vi "rqcAlice Key Distribution (Low Level Example).vi"() -> ()   [LabVIEW 2019]
uses:
  Custom Controls/rqcAlice States.ctl
  FPGA/Alice/Custom Controls/Phase Modulator/rqcAlice Mod.Config.ctl
  Shared/Shared FPGA Lib/Shared Logic/Custom Controls/rqc Random Generator.parameters.ctl
  Shared/Shared FPGA Lib/Shared Logic/Custom Controls/rqc Random Generator.value type.ctl
  FPGA/Alice/Custom Controls/Main State Machine/rqcAlice DAC Clock Positions.ctl
  Shared/Shared Host Lib/rqc ServiceNET/Custom Controls/rqc ServiceNET command.ctl
  Shared/Shared Host Lib/rqc ServiceNET/Alice/Custom Controls/rqcAlice ServiceNET control.ctl
  <vilib>/FPGAPlugInAG/PCIe-7820R/niLvFpga_Open_PCIe-7820R.vi
  <vilib>/rvi/interface/common/dynamic/niFpgaDynamicAddResources.vi
  <vilib>/FPGAPlugInAG/Dynamic/niLvFpga_Close_Dynamic.vi
  <vilib>/rvi/interface/nirviOpenFPGA/nirviOpenFPGA.xnode
  FPGA Bitfiles/rqcAlice FPGA (7820R) v 3.2.0.lvbitx
  <vilib>/rvi/interface/nirviCloseFPGA/nirviCloseFPGA.xnode
panel:
  in  "Attenuation, dB":dbl=10.0 max=40.0
  in  "Activate advanced parameters":bool
  in  "Sync mode":bool caption="«Coax / SD»"
  in  "PM RND":bool=TRUE caption="Alice's states randomisation"
  in  "Autoscale X":bool=TRUE caption="Show all QBER mesurements"
  out "QBER Graph":dbl(graph)=3.273809523809524
  out "IP Address":string="192.168.0.245" caption="Alice IP address"
  in  "DL SD":u32 caption="SD delay value"
  in  "pm.off":u8=1
  in  "pm.on":u8=9
  in  "Pi Voltage":u16=130
  out "Real pulse count:":i32=1000000 caption="Real sync pulses count:"
  out "Total pulses expected:":u32=1000000 caption="Sync pulses expected:"
  out "QBER, %":dbl=3.273809523809524
  out "Bob's Key:":string="010101101101101010110001010110000011111000011110110011101010000011100100011000000101000011010101100000000111001111111110010001000100001001000100101010000110100001001101001101100101111010101101000010110000010000000001000010001111000010111000011001111110111101100100010000011110101100100011100000100010001100000001100101100101001001100011001011010110001010010100111010111110001101000001001111101000001010001110011110101110100101011001101000000000101111011111010001001100001100110101000000100000010001001001011101101110100110111101000101110110001101011110011010001000111111101000100000011010000000000100..."
  out "Alice's Key:":string="010101101101101010110001010110000011111000011111110011101010000011100100100000000101000011010101100000000110001111110110000001000100001001000100001010100110100001001101001111100101111110101101000010110000010000000001000010001111000010111000011001111110111101100100010000011110101101100011100000100010001100000001100101100101001001100011001011010110001010010100111010111110101101000001001111101000001010001110011110100110100101011001101000000000101111011111010001001100001100110101000000100000010001001001011101001110000110111101000101110110000101011110011010001000111111101000100000011010000000000100..."
  in  "Pulses in Train":u32=1000 caption="Number of pulses in train"
  in  "Train Number":i32=1000 caption="Number of trains"
  in  "DL Coax":u32=23944 caption="Coax delay value"
  out "error out":errorcluster
  in  "Stop":bool
  out "Connection status":bool
  in  "Port":u16=5020
  out "Current State":T1=enum."App.Stop" caption="App current state"
  # "ALICE"
  # "LAN settings:"
  # "Sync pulses details:"
  # "«"
  # "»"
  # "Advanced\nPM parameters:\nRecommended \npm.on - [9]\npm.off - [1-2]"
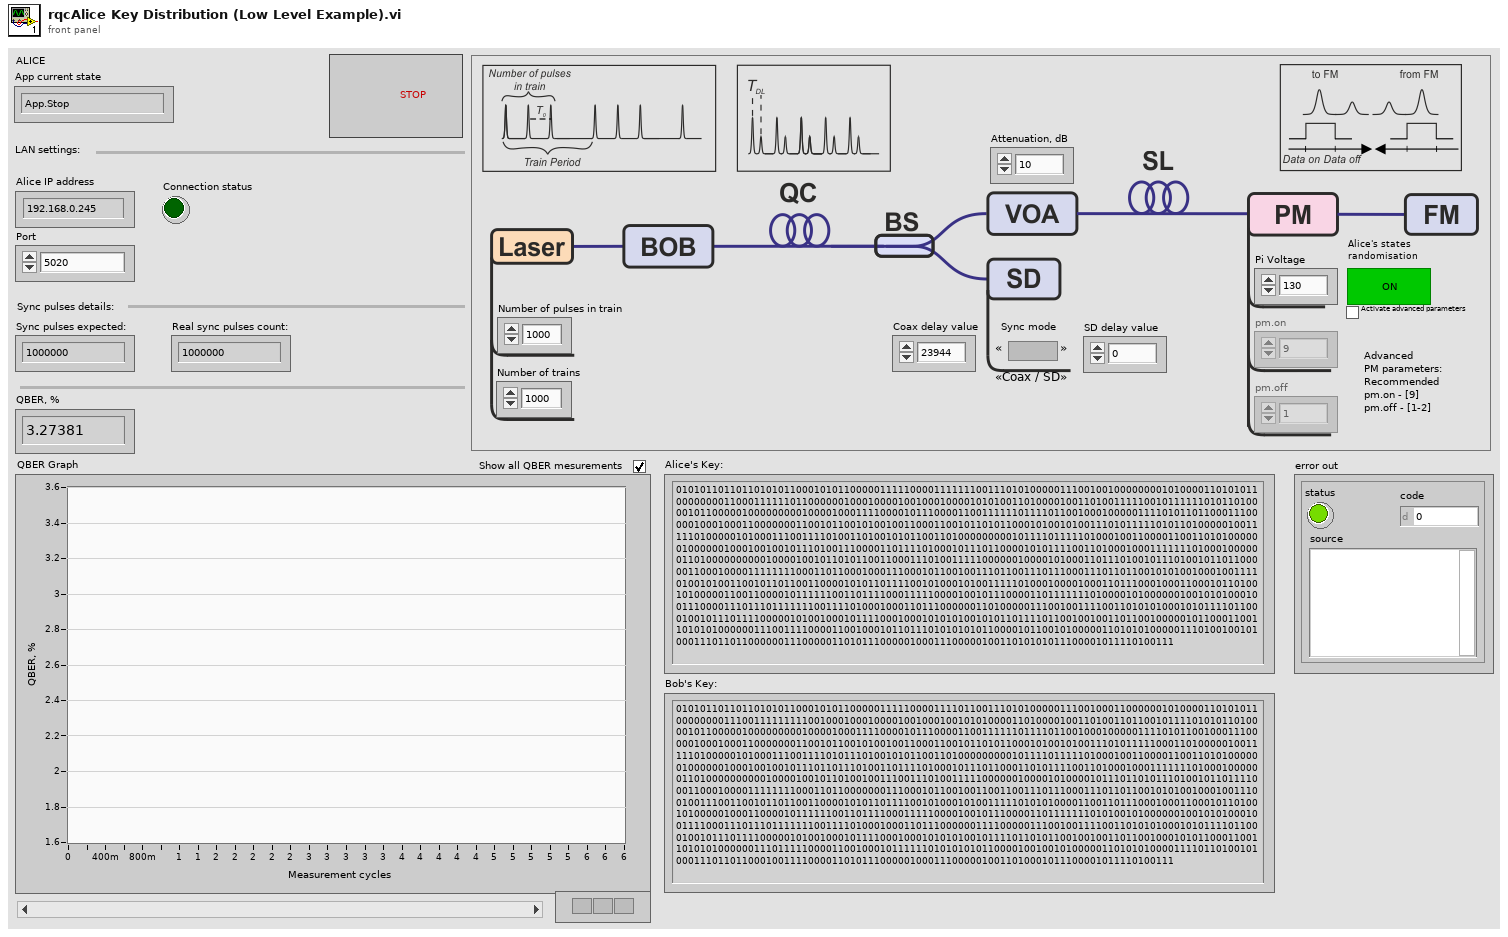
[diagram p1: front panel]
types:
  T1 = typedef "rqcAlice States.ctl" = enum16{"HW.configure", "HW.meas", "NET.create", "NET.connect", "NET.readCommand", "NET.sendCommand", "NET.readData", "NET.close", "Meas.Start", "Meas.NextStep", "Meas.restart", "Meas.Done", "App.HandleEvent", "App.HandleError", "App.Stop"}
  T2 = typedef "rqcAlice DAC Clock Positions.ctl" = u8[]
  T3 = typedef "rqc Random Generator.parameters.ctl" = cluster{"value type":T4, "constant":u16, "num of levels":u16, "levels values":u16[]}
  T4 = typedef "rqc Random Generator.value type.ctl" = enum32{"random value", "constant"}
  T5 = typedef "rqcAlice Mod.Config.ctl" = cluster{"mod.on":u8, "mod.off":u8}
  T6 = typedef "rqc ServiceNET command.ctl" = enum8{"NONE", "READY", "START", "PING"}
  T7 = enum16{"open", "replace", "create", "open or create", "replace or create", "replace or create with confirmation"}
  T8 = typedef "rqcAlice ServiceNET control.ctl" = cluster{"connection ID":refnum<k5>, "port":u16, "connected?":bool}
  T9 = enum8{"Enabled", "Disabled", "Disabled and Grayed Out"}
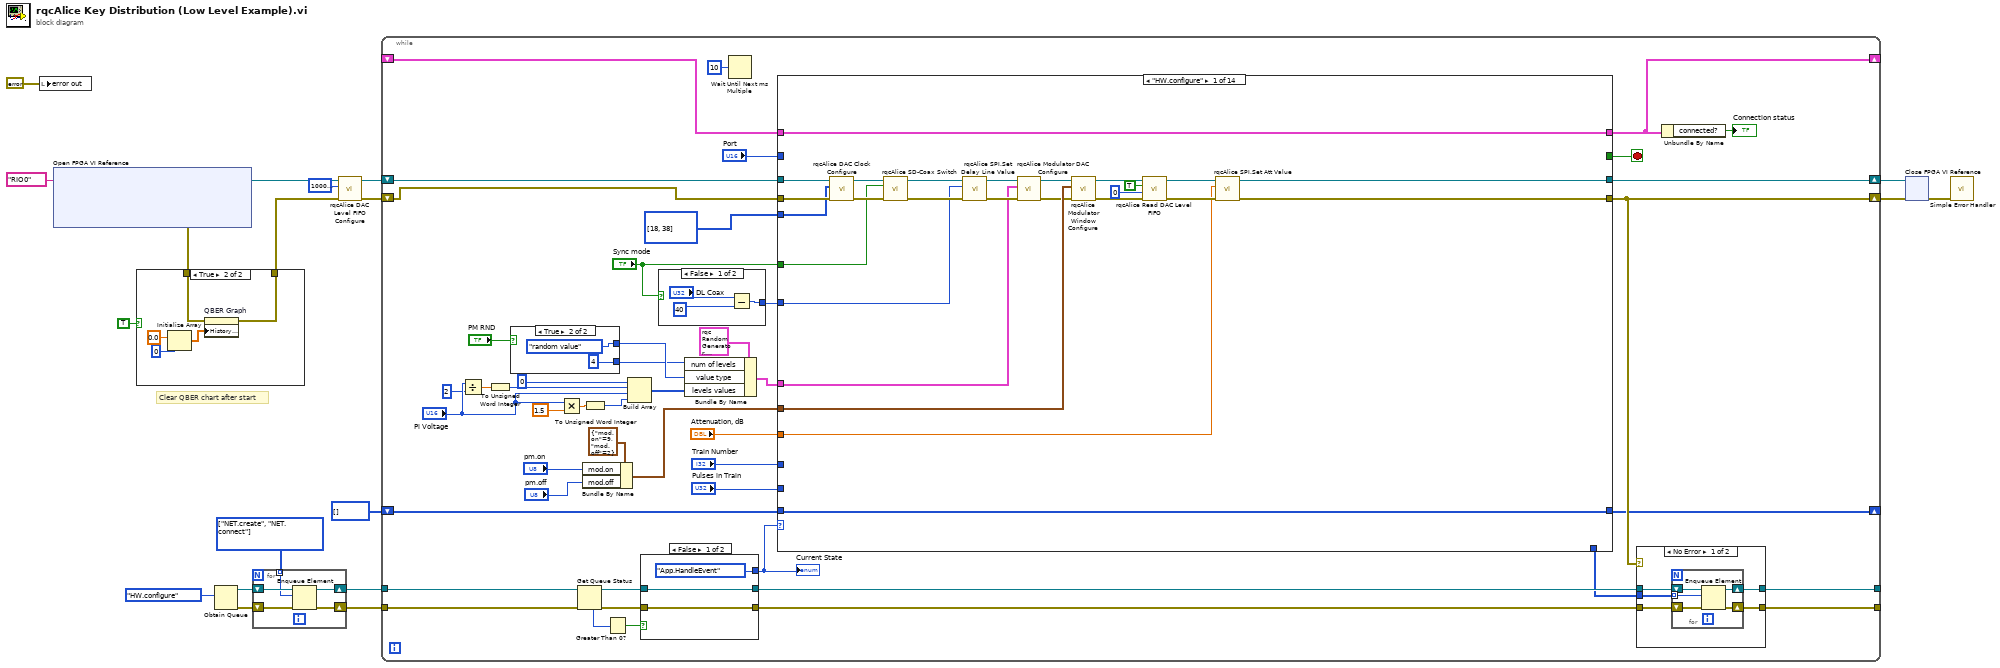
[diagram p0: block diagram]
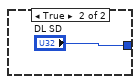
[diagram p3: hidden frame]
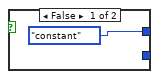
[diagram p4: hidden frame]
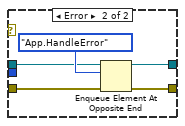
[diagram p5: hidden frame]
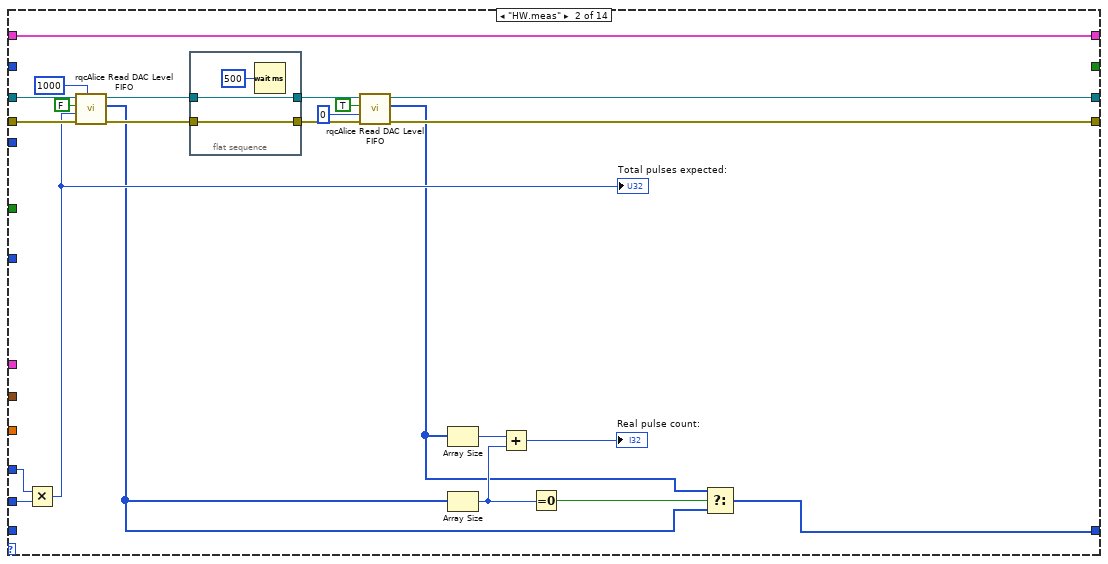
[diagram p6: hidden frame]
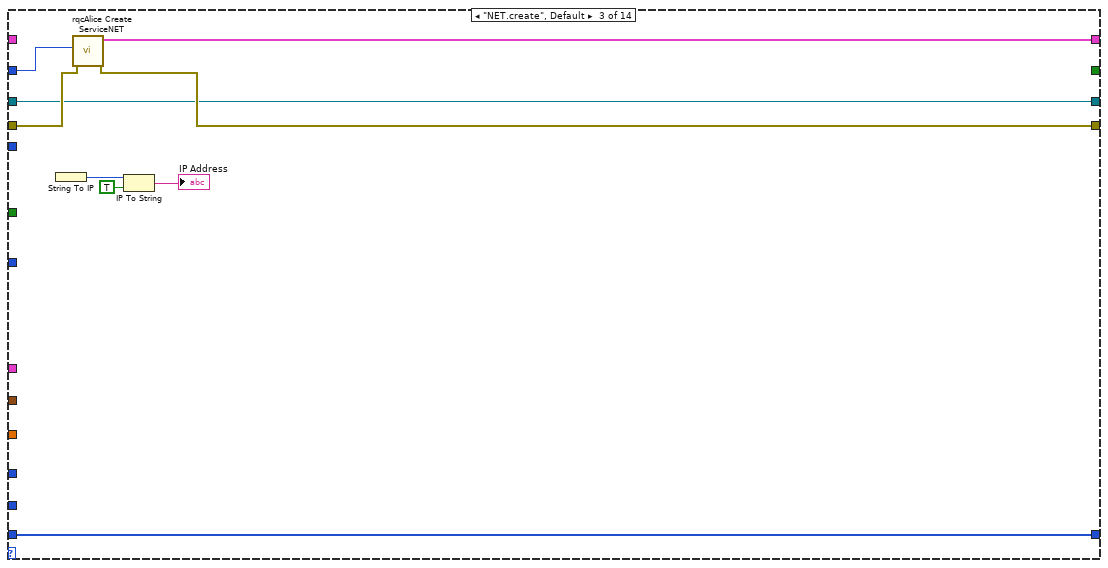
[diagram p7: hidden frame]
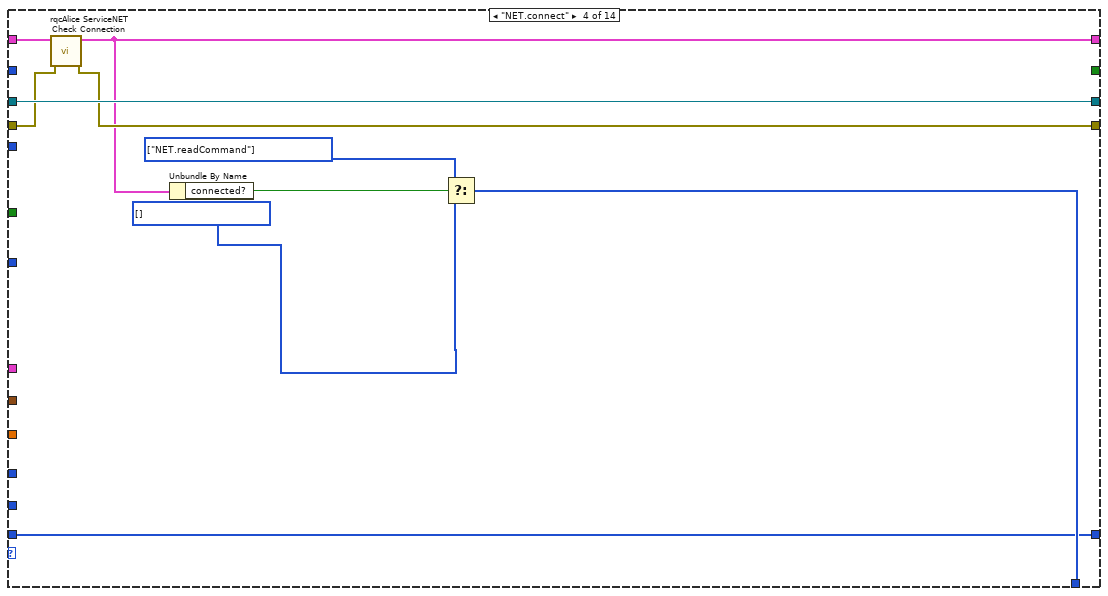
[diagram p8: hidden frame]
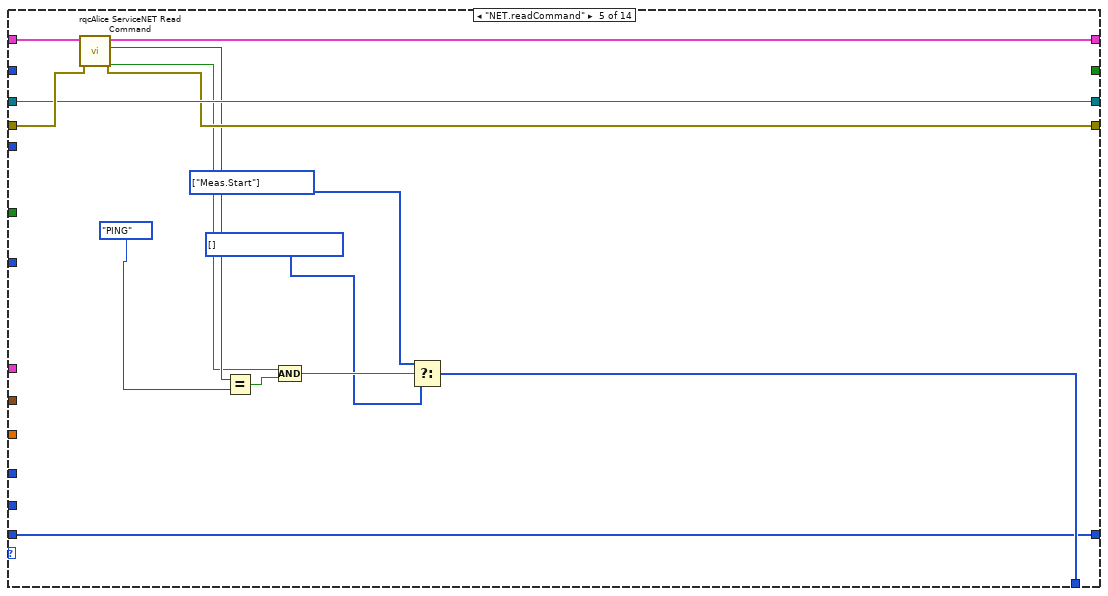
[diagram p9: hidden frame]
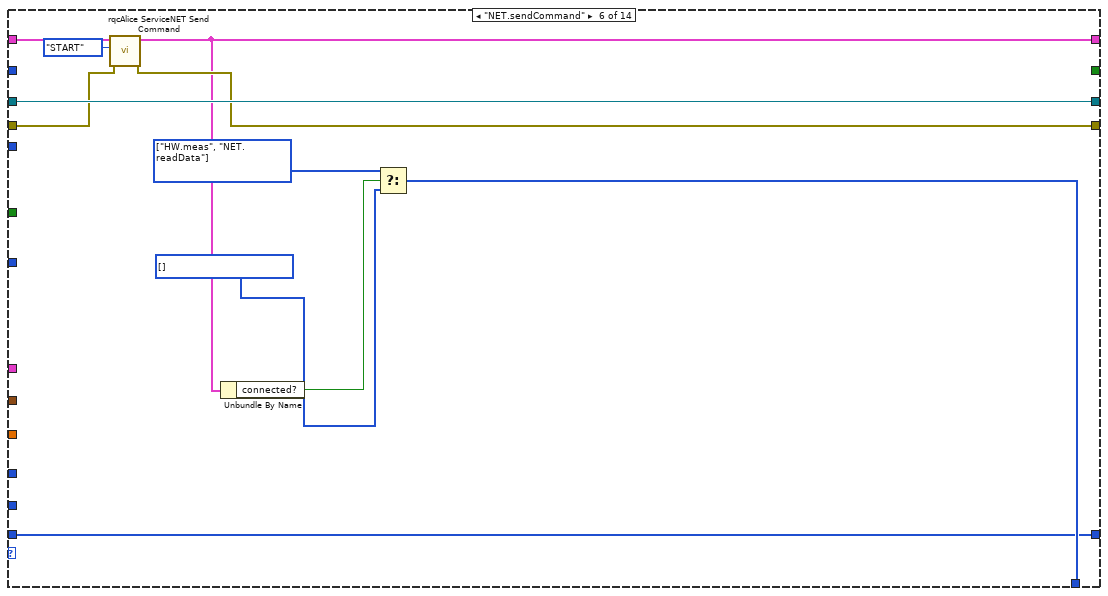
[diagram p10: hidden frame]
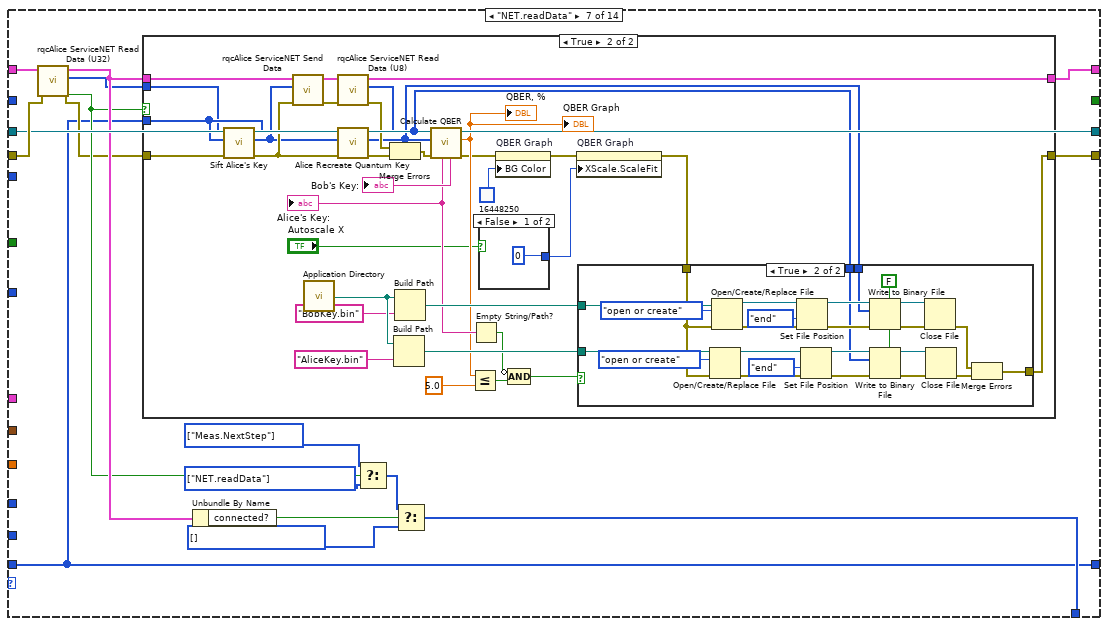
[diagram p11: hidden frame]
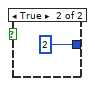
[diagram p13: hidden frame]
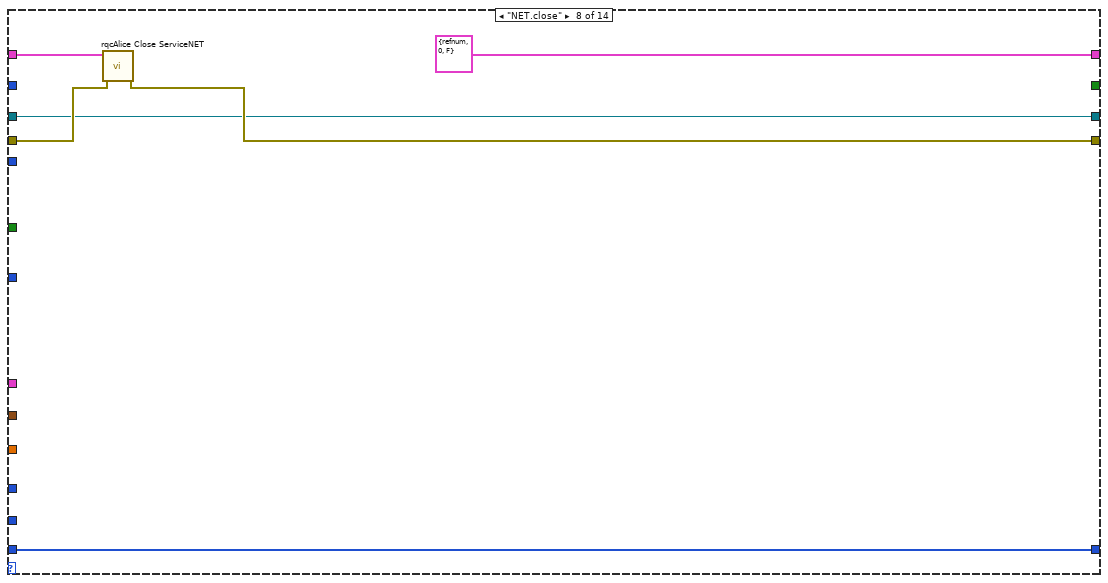
[diagram p15: hidden frame]
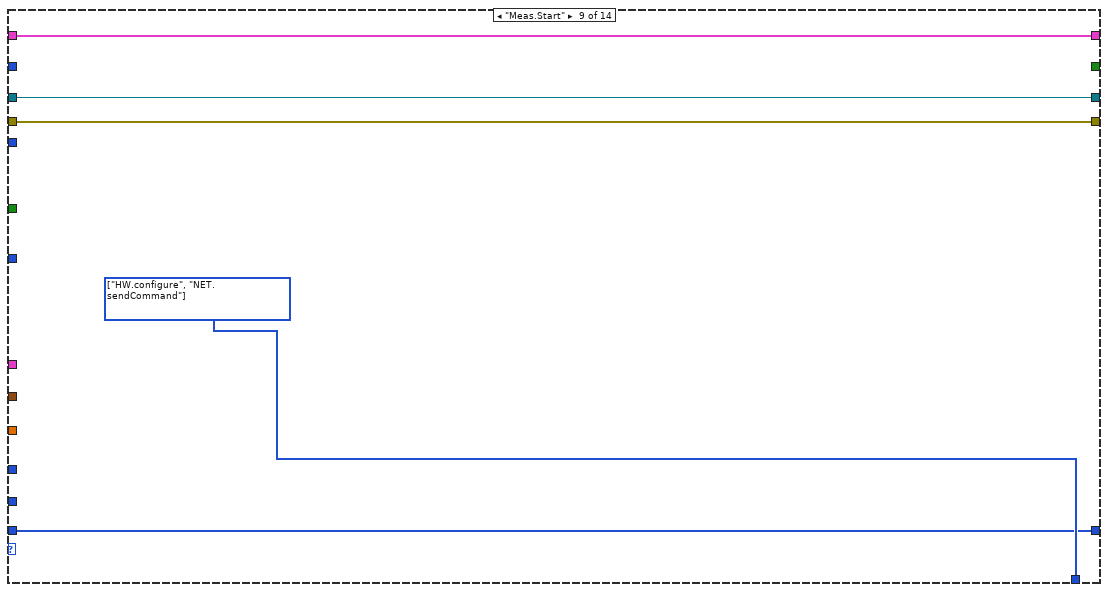
[diagram p16: hidden frame]
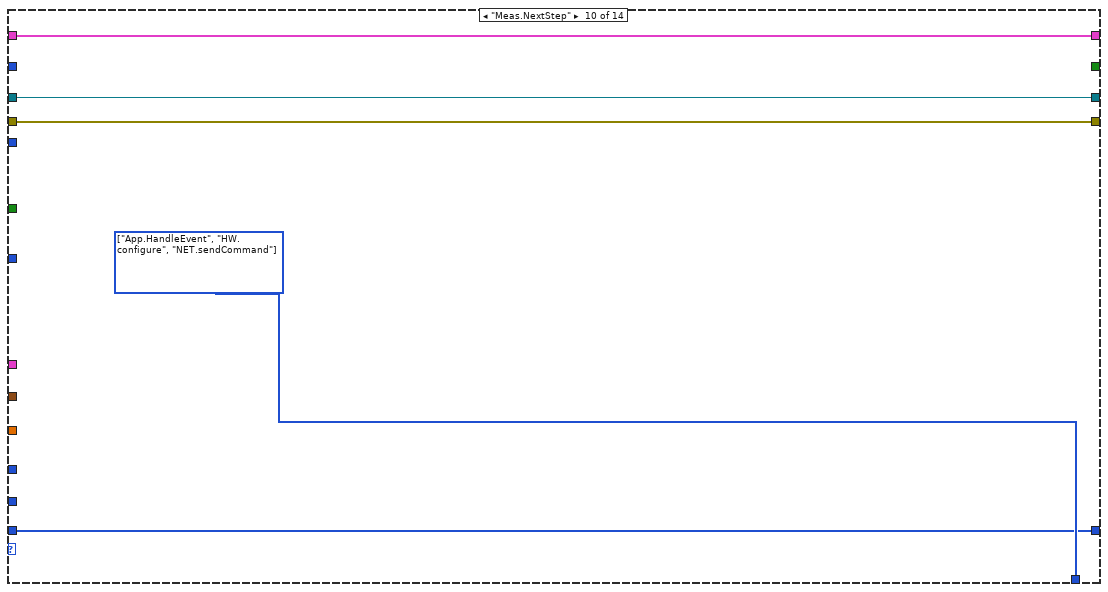
[diagram p17: hidden frame]
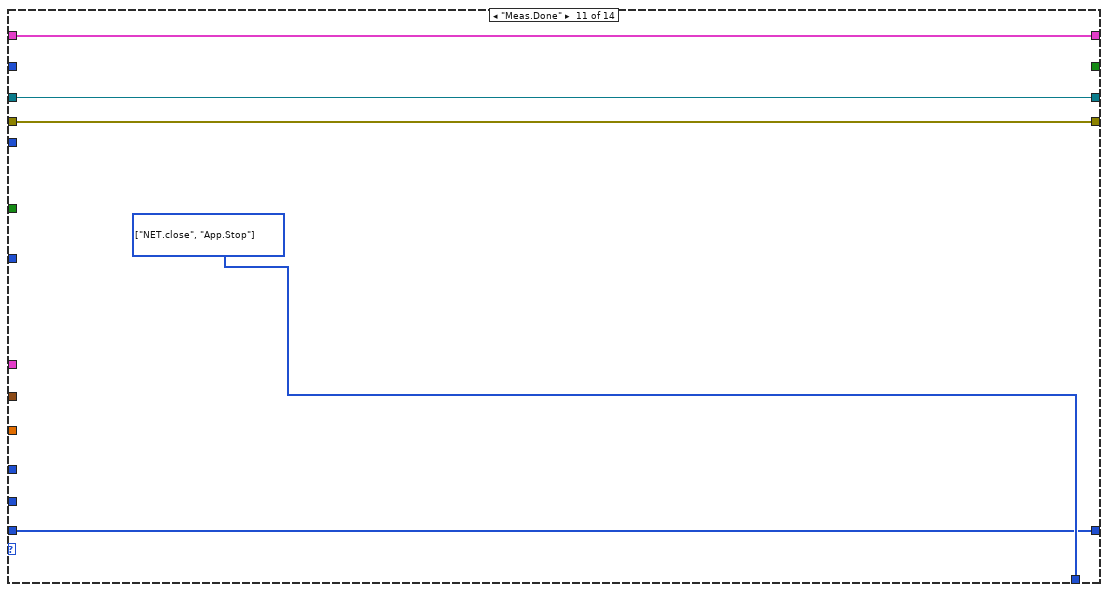
[diagram p18: hidden frame]
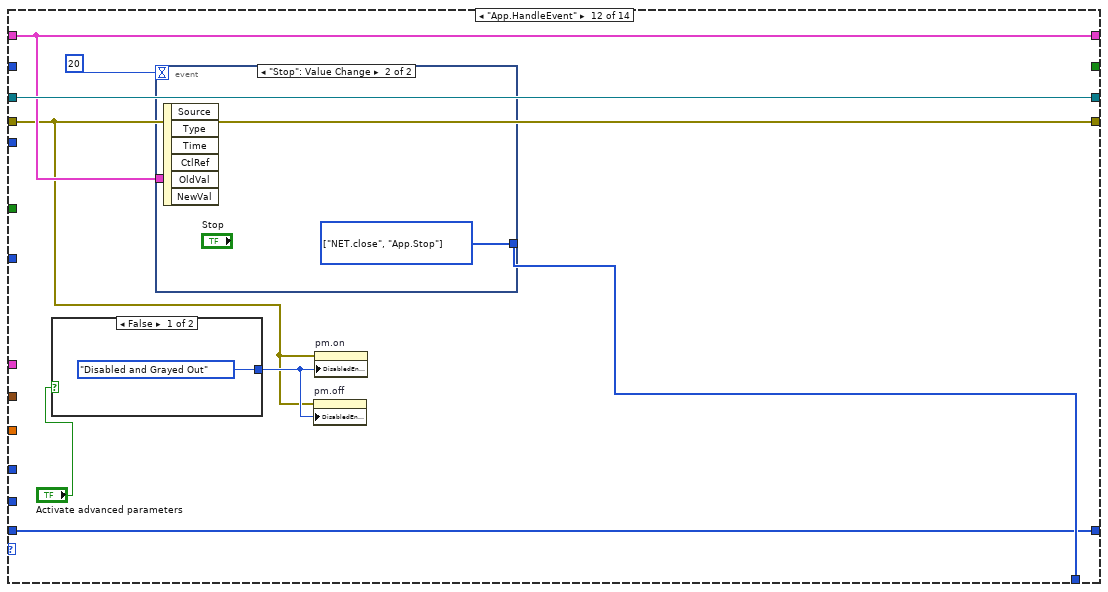
[diagram p19: hidden frame]
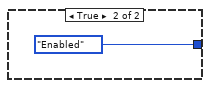
[diagram p20: hidden frame]
diagram:
  w13 = T1[] [enum."NET.create", enum."NET.connect"] items=["HW.configure", "HW.meas", "NET.create", "NET.connect", "NET.readCommand", "NET.sendCommand", "NET.readData", "NET.close", "Meas.Start", "Meas.NextStep", "Meas.restart", "Meas.Done", "App.HandleEvent", "App.HandleError", "App.Stop"]
  # "Clear QBER chart after start"
  n1 = local write "error out"(errorcluster {"status"=FALSE, "code"=0, "source"=""} ("error out")) -> ()
  n2 = xnode "Open FPGA VI Reference"("resource name"=tag "RIO0") -> ("FPGA VI Reference Out"=w8:refnum<k20>, "error out"=w3:errorcluster)  [unwired: 1 in]
  n3 = case shown="True" TRUE {
    tunnel: w3 -> [w20 w25]
    tunnel: [w20 w24] -> w2
    frame False {
    }
    frame True {
      n4 = Initialize Array(0.0 ("element"), 0 ("dimension size")) -> (w23:dbl[])
      n5 = property on="QBER Graph" class="WFChart (strict)"(error in=w25, "History Data"=w23) -> (error out=w24:errorcluster)  [unwired: 1 in, 1 out]
    }
  }
  n6 = Obtain Queue(element data type=rqcAlice_States."HW.configure" ("rqcAlice States")) -> (queue out=w15:refnum<queue>, error out=w14:errorcluster)  [unwired: 4 in, 1 out]
  n7 = for {
    shift-right: [w28] -> w12
    shift-left: w15 -> [w30]
    shift-right: [w27] -> w11
    shift-left: w14 -> [w29]
    tunnel: w13 -> [w26] mode=indexing
    n8 = Enqueue Element(queue=w30, element=w26, error in (no error)=w29) -> (queue out=w28:refnum<queue>, error out=w27:errorcluster)  [unwired: 1 in, 1 out]
  }
  n9 = call "rqcAlice DAC Level FIFO Configure.vi"("error in"=w2, "DAC Level FIFO Depth"=u32 10000000, "Alice FPGA Reference In"=w8) -> ("error out"=w6:errorcluster, "Alice FPGA Reference Out"=w7:refnum<k20>)  [unwired: 7 in]
  n10 = while {
    tunnel: w12 -> [w77]
    shift-right: [w78] -> w18
    shift-left: w7 -> [w41]
    shift-right: [w70] -> w17
    shift-left: w6 -> [w40]
    tunnel: w11 -> [w76]
    tunnel: [w67] -> _
    tunnel: [w66] -> _
    shift-right: [w62] -> _
    shift-left: _ -> [w64]
    shift-right: [w56] -> _
    shift-left: u8[] [] ("Data") -> [w55]
    stop <- w60 stop-if-true
    n11 = Divide(x="Pi Voltage", y=2) -> (x/y=w47:dbl)
    n12 = To Unsigned Word Integer(number=w47) -> (unsigned 16bit integer=w52:u16)
    n13 = case shown="True" "PM RND" {
      tunnel: [rqc_Random_Generator.value_type."constant" ("pm.value type") rqc_Random_Generator.value_type."random value" ("pm.value type")] -> w46
      tunnel: [_ u16 4 ("num of levels")] -> w33
      frame False {
      }
      frame True {
      }
    }
    n14 = Multiply(x="Pi Voltage", y=1.5) -> (x*y=w49:dbl)
    n15 = Get Queue Status(queue=w77, error in (no error)=w76) -> (queue out=w73:refnum<queue>, error out=w72:errorcluster, # elements in queue=w75:i32)  [unwired: 1 in, 5 out]
    n16 = Bundle By Name(cluster=T5 {"mod.on"=9, "mod.off"=2} ("Modulator config"), "mod.on"="pm.on", "mod.off"="pm.off") -> (w36:T5)
    n17 = To Unsigned Word Integer(number=w49) -> (unsigned 16bit integer=w54:u16)
    n18 = Greater Than 0?(x=w75) -> (x > 0?=w74:bool)
    n19 = Build Array(u16 0 ("element"), w52, "Pi Voltage", w54) -> (w45:u16[])
    n20 = case shown="False" w74 {
      tunnel: w73 -> [w325 w331]
      tunnel: w72 -> [w324 w330]
      tunnel: [rqcAlice_States."App.HandleEvent" ("rqcAlice States") w329] -> w71
      tunnel: [w325 w328] -> w69
      tunnel: [w324 w327] -> w68
      frame False {
      }
      frame True {
        n21 = Dequeue Element(queue=w331, error in (no error)=w330) -> (queue out=w328:refnum<queue>, element=w329:T1, error out=w327:errorcluster)  [unwired: 1 in, 1 out]
      }
    }
    "Current State" <- w71
    n22 = case shown="False" "Sync mode" {
      tunnel: [w81 "DL SD"] -> w42
      frame False {
        n23 = Subtract(x="DL Coax", y=40) -> (x-y=w81:u32)
      }
      frame True {
      }
    }
    n24 = Bundle By Name(cluster=T3 {"value type"=enum."random value", "constant"=150, "num of levels"=4, "levels values"=[0, 75, 150, 225]} ("RndGen.parameters"), "num of levels"=w33, "value type"=w46, "levels values"=w45) -> (w38:T3)
    n25 = Wait Until Next ms Multiple(millisecond multiple=u32 10) -> ()  [unwired: 1 out]
    n26 = case shown="\"HW.configure\"" w71 {
      tunnel: w41 -> [w126 w149 w158 w171 w182 w196 w210 w277 w285 w290 w295 w304 w317 w322]
      tunnel: w40 -> [w125 w148 w160 w169 w184 w194 w211 w280 w284 w289 w294 w298 w316 w321]
      tunnel: w36 -> [w124 _ _ _ _ _ _ _ _ _ _ _ _ _]
      tunnel: [w110 w141 w158 w171 w182 w196 w210 w277 w285 w290 w295 w304 w317 w322] -> w78
      tunnel: [w108 w140 w159 w168 w181 w193 w198 w279 w284 w289 w294 w298 errorcluster {"status"=FALSE, "code"=0, "source"=""} ("error out") w321] -> w70
      tunnel: [_ _ _ w164 w173 w187 w204 _ w283 w288 w293 w301 w314 _] -> w65
      tunnel: [w123 w144 w161 w167 w183 w191 w202 T8 {"connection ID"=refnum, "port"=0, "connected?"=FALSE} ("rqcAlice ServiceNET out") w286 w291 w296 w302 w318 w320] -> w62
      tunnel: w64 -> [w123 w144 _ w170 w185 w195 w212 w281 w286 w291 w296 w302 w318 w320]
      tunnel: "Port" -> [_ _ w157 _ _ _ _ _ _ _ _ _ _ _]
      tunnel: [_ _ _ _ _ _ _ _ _ _ _ _ _ TRUE] -> w60
      tunnel: w42 -> [w112 _ _ _ _ _ _ _ _ _ _ _ _ _]
      tunnel: "Train Number" -> [_ w147 _ _ _ _ _ _ _ _ _ _ _ _]
      tunnel: "Pulses in Train" -> [_ w146 _ _ _ _ _ _ _ _ _ _ _ _]
      tunnel: [w122 w131 w156 w162 w172 w186 w197 w276 w282 w287 w292 w300 w313 w319] -> w56
      tunnel: w55 -> [w122 _ w156 w162 w172 w186 w197 w276 w282 w287 w292 w300 w313 w319]
      tunnel: w38 -> [w104 _ _ _ _ _ _ _ _ _ _ _ _ _]
      tunnel: "Sync mode" -> [w115 _ _ _ _ _ _ _ _ _ _ _ _ _]
      tunnel: "Attenuation, dB" -> [w107 _ _ _ _ _ _ _ _ _ _ _ _ _]
      tunnel: T2 [18, 38] ("DAC Clock params") -> [w101 _ _ _ _ _ _ _ _ _ _ _ _ _]
      frame "HW.configure" {
        n27 = call "rqcAlice DAC Clock Configure.vi"("error in"=w125, "DAC Clock params"=w101, "Alice FPGA Reference In"=w126) -> ("error out"=w116:errorcluster, "Alice FPGA Reference Out"=w117:refnum<k20>)  [unwired: 7 in]
        n28 = call "rqcAlice SD-Coax Switch.vi"("error in"=w116, "SD/Coax Select"=w115, "Alice FPGA Reference In"=w117) -> ("error out"=w113:errorcluster, "Alice FPGA Reference Out"=w114:refnum<k20>)  [unwired: 7 in]
        n29 = call "rqcAlice SPI.Set Delay Line Value.vi"("error in"=w113, "Delay Line Value"=w112, "Alice FPGA Reference In"=w114) -> ("error out"=w105:errorcluster, "Alice FPGA Reference Out"=w106:refnum<k20>)  [unwired: 7 in]
        n30 = call "rqcAlice Modulator DAC Configure.vi"("error in"=w105, "RndGen.parameters"=w104, "Alice FPGA Reference In"=w106) -> ("error out"=w103:errorcluster, "Alice FPGA Reference Out"=w102:refnum<k20>)  [unwired: 7 in]
        n31 = call "rqcAlice Modulator Window Configure.vi"("error in"=w103, "Modulator config"=w124, "Alice FPGA Reference In"=w102) -> ("error out"=w119:errorcluster, "Alice FPGA Reference Out"=w118:refnum<k20>)  [unwired: 7 in]
        n32 = call "rqcAlice Read DAC Level FIFO.vi"("error in"=w119, "number of elements"=u32 0, "read all available"=TRUE, "Alice FPGA Reference In"=w118) -> ("error out"=w109:errorcluster, "Alice FPGA Reference Out"=w111:refnum<k20>)  [unwired: 4 in, 2 out]
        n33 = call "rqcAlice SPI.Set Att Value.vi"("error in"=w109, "Attenuation, dB"=w107, "Alice FPGA Reference In"=w111) -> ("error out"=w108:errorcluster, "Alice FPGA Reference Out"=w110:refnum<k20>)  [unwired: 7 in]
      }
      frame "HW.meas" {
        n34 = Multiply(x=w147, y=w146) -> (x*y=w143:u32)
        "Total pulses expected:" <- w143
        n35 = call "rqcAlice Read DAC Level FIFO.vi"("timeout (ms)"=1000, "error in"=w148, "number of elements"=w143, "read all available"=FALSE, "Alice FPGA Reference In"=w149) -> ("error out"=w137:errorcluster, "Data"=w135:u8[], "Alice FPGA Reference Out"=w136:refnum<k20>)  [unwired: 3 in, 1 out]
        n36 = flat-sequence {
          tunnel: [w152] -> w128
          tunnel: w137 -> [w152]
          tunnel: [w151] -> w127
          tunnel: w136 -> [w151]
          frame #0 {
            n37 = Wait (ms)(milliseconds to wait=u32 500) -> ()  [unwired: 1 out]
          }
        }
        n38 = call "rqcAlice Read DAC Level FIFO.vi"("error in"=w128, "number of elements"=u32 0, "read all available"=TRUE, "Alice FPGA Reference In"=w127) -> ("error out"=w140:errorcluster, "Data"=w132:u8[], "Alice FPGA Reference Out"=w141:refnum<k20>)  [unwired: 4 in, 1 out]
        n39 = Array Size(array=w132) -> (size(s)=w138:i32)
        n40 = Array Size(array=w135) -> (size(s)=w134:i32)
        n41 = Add(x=w138, y=w134) -> (x+y=→"Real pulse count:":i32)
        n42 = Equal To 0?(x=w134) -> (x = 0?=w133:bool)
        n43 = Select(t=w132, s=w133, f=w135) -> (s? t:f=w131:u8[])
      }
      frame "NET.create", Default {
        n44 = String To IP() -> (0:w154:u32)  [unwired: 1 in]
        n45 = call "rqcAlice Create ServiceNET.vi"("error in"=w160, "port"=w157) -> ("error out"=w159:errorcluster, "rqcAlice ServiceNET control"=w161:T8)  [unwired: 8 in]
        n46 = IP To String(1:TRUE ("dot notation? (F)"), 2:w154) -> (0:→"IP Address":string)
      }
      frame "NET.connect" {
        w163 = T1[] [] items=["HW.configure", "HW.meas", "NET.create", "NET.connect", "NET.readCommand", "NET.sendCommand", "NET.readData", "NET.close", "Meas.Start", "Meas.NextStep", "Meas.restart", "Meas.Done", "App.HandleEvent", "App.HandleError", "App.Stop"] ("f")
        w165 = T1[] [enum."NET.readCommand"] items=["HW.configure", "HW.meas", "NET.create", "NET.connect", "NET.readCommand", "NET.sendCommand", "NET.readData", "NET.close", "Meas.Start", "Meas.NextStep", "Meas.restart", "Meas.Done", "App.HandleEvent", "App.HandleError", "App.Stop"]
        n47 = call "rqcAlice ServiceNET Check Connection.vi"("error in"=w169, "rqcAlice ServiceNET in"=w170) -> ("error out"=w168:errorcluster, "rqcAlice ServiceNET out"=w167:T8)  [unwired: 8 in]
        n48 = Unbundle By Name(w167) -> ("connected?"=w166:bool)
        n49 = Select(t=w165, s=w166, f=w163) -> (s? t:f=w164:T1[])
      }
      frame "NET.readCommand" {
        w174 = T1[] [] items=["HW.configure", "HW.meas", "NET.create", "NET.connect", "NET.readCommand", "NET.sendCommand", "NET.readData", "NET.close", "Meas.Start", "Meas.NextStep", "Meas.restart", "Meas.Done", "App.HandleEvent", "App.HandleError", "App.Stop"] ("f")
        w175 = T1[] [enum."Meas.Start"] items=["HW.configure", "HW.meas", "NET.create", "NET.connect", "NET.readCommand", "NET.sendCommand", "NET.readData", "NET.close", "Meas.Start", "Meas.NextStep", "Meas.restart", "Meas.Done", "App.HandleEvent", "App.HandleError", "App.Stop"] ("f")
        n50 = call "rqcAlice ServiceNET Read Command.vi"("error in"=w184, "rqcAlice ServiceNET in"=w185) -> ("error out"=w181:errorcluster, "cmd valid"=w177:bool, "command"=w179:T6, "rqcAlice ServiceNET out"=w183:T8)  [unwired: 6 in]
        n51 = Equal?(x=w179, y=rqc_ServiceNET_command."PING" ("command")) -> (x = y?=w178:bool)
        n52 = Compound Arithmetic op=AND(w177, w178) -> (w176:bool)
        n53 = Select(t=w175, s=w176, f=w174) -> (s? t:f=w173:T1[])
      }
      frame "NET.sendCommand" {
        w188 = T1[] [] items=["HW.configure", "HW.meas", "NET.create", "NET.connect", "NET.readCommand", "NET.sendCommand", "NET.readData", "NET.close", "Meas.Start", "Meas.NextStep", "Meas.restart", "Meas.Done", "App.HandleEvent", "App.HandleError", "App.Stop"] ("f")
        w189 = T1[] [enum."HW.meas", enum."NET.readData"] items=["HW.configure", "HW.meas", "NET.create", "NET.connect", "NET.readCommand", "NET.sendCommand", "NET.readData", "NET.close", "Meas.Start", "Meas.NextStep", "Meas.restart", "Meas.Done", "App.HandleEvent", "App.HandleError", "App.Stop"] ("f")
        n54 = call "rqcAlice ServiceNET Send Command.vi"("error in"=w194, "command"=rqc_ServiceNET_command."START", "rqcAlice ServiceNET in"=w195) -> ("error out"=w193:errorcluster, "rqcAlice ServiceNET out"=w191:T8)  [unwired: 7 in]
        n55 = Unbundle By Name(w191) -> ("connected?"=w190:bool)
        n56 = Select(t=w189, s=w190, f=w188) -> (s? t:f=w187:T1[])
      }
      frame "NET.readData" {
        w205 = T1[] [] items=["HW.configure", "HW.meas", "NET.create", "NET.connect", "NET.readCommand", "NET.sendCommand", "NET.readData", "NET.close", "Meas.Start", "Meas.NextStep", "Meas.restart", "Meas.Done", "App.HandleEvent", "App.HandleError", "App.Stop"] ("f")
        w209 = T1[] [enum."Meas.NextStep"] items=["HW.configure", "HW.meas", "NET.create", "NET.connect", "NET.readCommand", "NET.sendCommand", "NET.readData", "NET.close", "Meas.Start", "Meas.NextStep", "Meas.restart", "Meas.Done", "App.HandleEvent", "App.HandleError", "App.Stop"] ("t")
        w208 = T1[] [enum."NET.readData"] items=["HW.configure", "HW.meas", "NET.create", "NET.connect", "NET.readCommand", "NET.sendCommand", "NET.readData", "NET.close", "Meas.Start", "Meas.NextStep", "Meas.restart", "Meas.Done", "App.HandleEvent", "App.HandleError", "App.Stop"] ("f")
        n57 = call "rqcAlice ServiceNET Read Data (U32).vi"("error in"=w211, "rqcAlice ServiceNET in"=w212) -> ("error out"=w200:errorcluster, "data valid"=w201:bool, "data"=w199:u32[], "rqcAlice ServiceNET out"=w203:T8)  [unwired: 6 in]
        n58 = case shown="True" w201 {
          tunnel: [w214 w243] -> w202
          tunnel: w203 -> [w214 w246]
          tunnel: w200 -> [w213 w247]
          tunnel: w199 -> [_ w237]
          tunnel: w197 -> [_ w242]
          tunnel: [w213 w229] -> w198
          frame False {
          }
          frame True {
            n59 = call "Sift Alice's Key.vi"("error in"=w247, "Alice's Raw Data in"=w242, "Bob's Data in"=w237) -> ("error out"=w241:errorcluster, "Bob's correct measurements indexes"=w236:u32[])  [unwired: 6 in, 1 out]
            n60 = call "rqcAlice ServiceNET Send Data.vi"("error in"=w241, "Data"=w236, "rqcAlice ServiceNET in"=w246) -> ("error out"=w244:errorcluster, "rqcAlice ServiceNET out"=w245:T8)  [unwired: 7 in]
            n61 = call <vilib>:"Application Directory.vi"() -> ("Application Directory"=w235:path)
            n62 = call "rqcAlice ServiceNET Read Data (U8).vi"("error in"=w244, "rqcAlice ServiceNET in"=w245) -> ("error out"=w238:errorcluster, "data"=w222:u8[], "rqcAlice ServiceNET out"=w243:T8)  [unwired: 6 in, 1 out]
            n63 = call "Alice Recreate Quantum Key.vi"("error in"=w241, "Correct Measurements Indexes in"=w236, "Raw Data in"=w242) -> ("error out"=w240:errorcluster, "Sifted Key out"=w223:u8[])  [unwired: 6 in, 1 out]
            n64 = Merge Errors(w238, w240) -> (w239:errorcluster)
            n65 = Build Path(base path=w235, name or relative path="AliceKey.bin") -> (appended path=w231:path)
            n66 = Build Path(base path=w235, name or relative path="BobKey.bin") -> (appended path=w232:path)
            n67 = call "Calculate QBER.vi"("error in"=w239, "Alice's Key"=w223, "Bob's Key"=w222) -> ("error out"=w219:errorcluster, "QBER, %"=w221:dbl, "Bob's Key:"=→"Bob's Key:":string, "Alice's Key:"=w226:string)  [unwired: 5 in]
            "Alice's Key:" <- w226
            "QBER, %" <- w221
            "QBER Graph" <- w221
            n68 = Less Or Equal?(x=w221, y=5.0) -> (x <= y?=w228:bool)
            n69 = Empty String/Path?(string/path=w226) -> (empty?=w224:bool)
            n70 = case shown="False" "Autoscale X" {
              tunnel: [u8 0 u8 2] -> w216
              frame False {
              }
              frame True {
              }
            }
            n71 = property on="QBER Graph" class="WFChart (strict)"(error in=w219, "BG Color"=u32 16448250) -> (error out=w217:errorcluster)  [unwired: 1 in, 1 out]
            n72 = Compound Arithmetic op=AND(invert w224, w228) -> (w225:bool)
            n73 = property on="QBER Graph" class="WFChart (strict)"(error in=w217, "XScale.ScaleFit"=w216) -> (error out=w218:errorcluster)  [unwired: 1 in, 1 out]
            n74 = case shown="True" w225 {
              tunnel: w232 -> [_ w275]
              tunnel: w231 -> [_ w272]
              tunnel: w218 -> [w250 w271]
              tunnel: [w250 w264] -> w229
              tunnel: w223 -> [_ w252]
              tunnel: w222 -> [_ w251]
              frame False {
              }
              frame True {
                w263 = FALSE ("prepend array or string size? (T)")
                n75 = Open/Create/Replace File(file path (use dialog)=w272, error in=w271, operation (0:open)=T7."open or create") -> (refnum out=w257:refnum<file>, error out=w253:errorcluster)  [unwired: 3 in, 1 out]
                n76 = Open/Create/Replace File(file path (use dialog)=w275, error in=w271, operation (0:open)=T7."open or create") -> (refnum out=w262:refnum<file>, error out=w260:errorcluster)  [unwired: 3 in, 1 out]
                n77 = Set File Position(refnum=w262, from (0:start)=enum16{"start", "end", "current"}."end", error in=w260) -> (refnum out=w261:refnum<file>, error out=w259:errorcluster)  [unwired: 1 in]
                n78 = Set File Position(refnum=w257, from (0:start)=enum16{"start", "end", "current"}."end", error in=w253) -> (refnum out=w256:refnum<file>, error out=w254:errorcluster)  [unwired: 1 in]
                n79 = Write to Binary File(file (use dialog)=w261, data=w252, error in=w259, 5:w263) -> (refnum out=w270:refnum<file>, error out=w269:errorcluster)  [unwired: 2 in, 1 out]
                n80 = Write to Binary File(file (use dialog)=w256, data=w251, error in=w254, 5:w263) -> (refnum out=w268:refnum<file>, error out=w267:errorcluster)  [unwired: 2 in, 1 out]
                n81 = Close File(refnum=w270, error in=w269) -> (error out=w266:errorcluster)  [unwired: 1 out]
                n82 = Close File(refnum=w268, error in=w267) -> (error out=w265:errorcluster)  [unwired: 1 out]
                n83 = Merge Errors(w266, w265) -> (w264:errorcluster)
              }
            }
          }
        }
        n84 = Unbundle By Name(w203) -> ("connected?"=w207:bool)
        n85 = Select(t=w209, s=w201, f=w208) -> (s? t:f=w206:T1[])
        n86 = Select(t=w206, s=w207, f=w205) -> (s? t:f=w204:T1[])
      }
      frame "NET.close" {
        n87 = call "rqcAlice Close ServiceNET.vi"("error in"=w280, "rqcAlice ServiceNET in"=w281) -> ("error out"=w279:errorcluster)  [unwired: 9 in]
      }
      frame "Meas.Start" {
        w283 = T1[] [enum."HW.configure", enum."NET.sendCommand"] items=["HW.configure", "HW.meas", "NET.create", "NET.connect", "NET.readCommand", "NET.sendCommand", "NET.readData", "NET.close", "Meas.Start", "Meas.NextStep", "Meas.restart", "Meas.Done", "App.HandleEvent", "App.HandleError", "App.Stop"] ("f")
      }
      frame "Meas.NextStep" {
        w288 = T1[] [enum."App.HandleEvent", enum."HW.configure", enum."NET.sendCommand"] items=["HW.configure", "HW.meas", "NET.create", "NET.connect", "NET.readCommand", "NET.sendCommand", "NET.readData", "NET.close", "Meas.Start", "Meas.NextStep", "Meas.restart", "Meas.Done", "App.HandleEvent", "App.HandleError", "App.Stop"] ("f")
      }
      frame "Meas.Done" {
        w293 = T1[] [enum."NET.close", enum."App.Stop"] items=["HW.configure", "HW.meas", "NET.create", "NET.connect", "NET.readCommand", "NET.sendCommand", "NET.readData", "NET.close", "Meas.Start", "Meas.NextStep", "Meas.restart", "Meas.Done", "App.HandleEvent", "App.HandleError", "App.Stop"] ("f")
      }
      frame "App.HandleEvent" {
        n88 = case shown="False" "Activate advanced parameters" {
          tunnel: [T9."Disabled and Grayed Out" ("Disabled") T9."Enabled" ("Disabled")] -> w299
          frame False {
          }
          frame True {
          }
        }
        n89 = event shown="[1] \"Stop\": Value Change" {
          selector: _ -> [_ _]
          dyn-events: _ -> [_ _]
          timeout: 20 -> [_ _]
          tunnel: w302 -> [w311 _]
          tunnel: [w307 w312] -> w301
          event Timeout {
            w308 = T1[] [enum."NET.create", enum."NET.connect"] items=["HW.configure", "HW.meas", "NET.create", "NET.connect", "NET.readCommand", "NET.sendCommand", "NET.readData", "NET.close", "Meas.Start", "Meas.NextStep", "Meas.restart", "Meas.Done", "App.HandleEvent", "App.HandleError", "App.Stop"]
            w309 = T1[] [] items=["HW.configure", "HW.meas", "NET.create", "NET.connect", "NET.readCommand", "NET.sendCommand", "NET.readData", "NET.close", "Meas.Start", "Meas.NextStep", "Meas.restart", "Meas.Done", "App.HandleEvent", "App.HandleError", "App.Stop"]
            n90 = event-data() -> ()  [unwired: 1 in, 3 out]
            n91 = Unbundle By Name(w311) -> ("connected?"=w310:bool)
            n92 = Select(t=w309, s=w310, f=w308) -> (s? t:f=w307:T1[])
          }
          event "Stop": Value Change {
            w312 = T1[] [enum."NET.close", enum."App.Stop"] items=["HW.configure", "HW.meas", "NET.create", "NET.connect", "NET.readCommand", "NET.sendCommand", "NET.readData", "NET.close", "Meas.Start", "Meas.NextStep", "Meas.restart", "Meas.Done", "App.HandleEvent", "App.HandleError", "App.Stop"]
            n93 = event-data() -> ()  [unwired: 1 in, 6 out]
          }
        }
        n94 = property on="pm.off" class="DigNum (strict)"(error in=w298, "DisabledEnum"=w299) -> ()  [unwired: 1 in, 2 out]
        n95 = property on="pm.on" class="DigNum (strict)"(error in=w298, "DisabledEnum"=w299) -> ()  [unwired: 1 in, 2 out]
      }
      frame "App.HandleError" {
        w314 = T1[] [enum."NET.close", enum."App.Stop"] items=["HW.configure", "HW.meas", "NET.create", "NET.connect", "NET.readCommand", "NET.sendCommand", "NET.readData", "NET.close", "Meas.Start", "Meas.NextStep", "Meas.restart", "Meas.Done", "App.HandleEvent", "App.HandleError", "App.Stop"] ("f")
        "error out" <- w316
      }
      frame "App.Stop" {
      }
    }
    n96 = case shown="No Error" w70 {
      tunnel: w69 -> [w90 w99]
      tunnel: w68 -> [w89 w97]
      tunnel: [w88 w98] -> w67
      tunnel: [w87 w96] -> w66
      tunnel: w65 -> [w86 _]
      frame No Error {
        n97 = for {
          shift-right: [w93] -> w88
          shift-left: w90 -> [w95]
          shift-right: [w92] -> w87
          shift-left: w89 -> [w94]
          tunnel: w86 -> [w91] mode=indexing
          n98 = Enqueue Element(queue=w95, element=w91, error in (no error)=w94) -> (queue out=w93:refnum<queue>, error out=w92:errorcluster)  [unwired: 1 in, 1 out]
        }
      }
      frame Error {
        n99 = Enqueue Element At Opposite End(queue=w99, element=rqcAlice_States."App.HandleError" ("rqcAlice States"), error in (no error)=w97) -> (queue out=w98:refnum<queue>, error out=w96:errorcluster)  [unwired: 1 in, 1 out]
      }
    }
    n100 = Unbundle By Name(w62) -> ("connected?"=→"Connection status":bool)
  }
  n101 = xnode "Close FPGA VI Reference"("FPGA VI Reference In"=w18, "error in"=w17) -> ("error out"=w10:errorcluster)
  n102 = call <vilib>:"Simple Error Handler.vi"("error in (no error)"=w10) -> ()  [unwired: 4 in, 5 out]
